vi "getAxialPaths.vi"(11 "platform":i32) -> (1 "platform indices":i32[](array[numeric]), 3 "paths through start":dbl[][](array[numeric]))   [LabVIEW 2017]
panel:
  out "all rows":dbl[][](array[numeric])
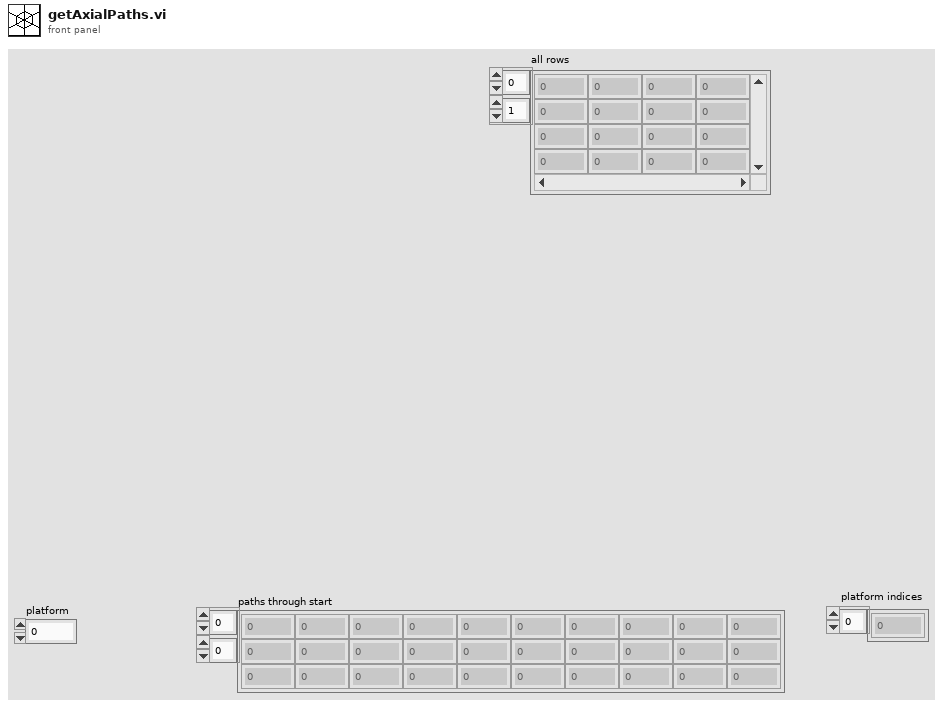
[diagram p1: front panel]
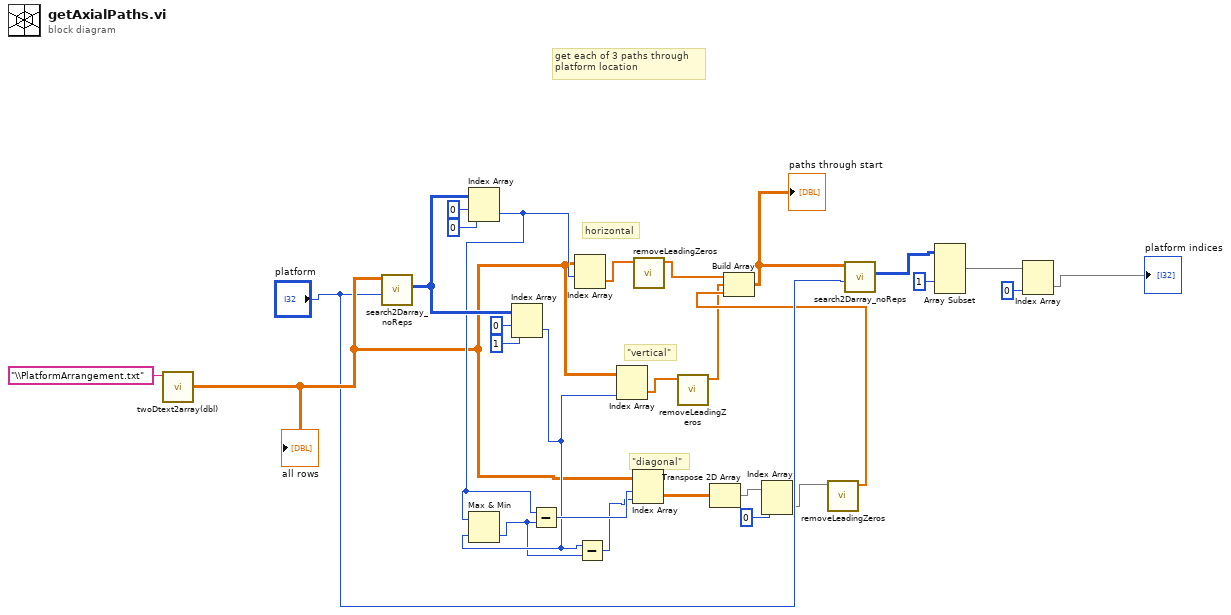
[diagram p0: block diagram]
diagram:
  # "\"diagonal\""
  # "\"vertical\""
  # "horizontal"
  # "get each of 3 paths through \nplatform location"
  n1 = call "twoDtext2array(dbl).vi"("String"="\\PlatformArrangement.txt") -> ("all rows"=w16:dbl[][])  [unwired: 10 in]
  "all rows" <- w16
  n2 = call "search2Darray_noReps.vi"("target"="platform", "Array"=w16) -> ("indices"=w25:i32[][])  [unwired: 9 in]
  n3 = Index Array(array=w25, index (row)=0, index (col)=0 ("disabled index (col)")) -> (element=w21:i32)
  n4 = Index Array(array=w25, index (row)=0, index (col)=1 ("disabled index (col)")) -> (element=w19:i32)
  n5 = Max & Min(x=w21, y=w19) -> (min(x,y)=w18:i32)  [unwired: 1 out]
  n6 = Subtract(x=w21, y=w18) -> (x-y=w20:i32)
  n7 = Index Array(array=w16, index (row)=w21) -> (element=w2:dbl[])  [unwired: 1 in]
  n8 = Subtract(x=w19, y=w18) -> (x-y=w17:i32)
  n9 = Index Array(array=w16, index (col)=w19) -> (element=w4:dbl[])  [unwired: 1 in]
  n10 = Index Array(array=w16, index (row)=w20, index (col)=w17) -> (element=w22:dbl[][])
  n11 = call "removeLeadingZeros.vi"("input"=w2) -> ("output"=w1:dbl[])  [unwired: 10 in]
  n12 = call "removeLeadingZeros.vi"("input"=w4) -> ("output"=w3:dbl[])  [unwired: 10 in]
  n13 = Transpose 2D Array(2D array=w22) -> (transposed array=w8:dbl[][])
  n14 = Index Array(array=w8, index (row)=0) -> (element=w6:dbl[])  [unwired: 1 in]
  n15 = call "removeLeadingZeros.vi"("input"=w6) -> ("output"=w5:dbl[])  [unwired: 10 in]
  n16 = Build Array(w1, w3, w5) -> (w15:dbl[][])
  "paths through start" <- w15
  n17 = call "search2Darray_noReps.vi"("target"="platform", "Array"=w15) -> ("indices"=w13:i32[][])  [unwired: 9 in]
  n18 = Array Subset(array=w13, index (col)=1 ("index")) -> (w11:i32[][])  [unwired: 3 in]
  n19 = Index Array(array=w11, index (col)=0 ("disabled index (col)")) -> (element=→"platform indices":i32[])  [unwired: 1 in]
